vi "FPGA_1R_ADC_1W_DAC_2AI_Jul9.vi"() -> ()   [LabVIEW 2019]
uses:
  <vilib>/rvi/Emulation/niFpgaGetClockAttributes.vi
  <vilib>/rvi/Emulation/niFpgaSctlEmulationGetInTimedLoop.vi
  <vilib>/rvi/Emulation/niFpgaEmulationReportErrorSimple.vi
  <vilib>/rvi/eio/common/nirviEmuTemplateMethod_errors.vi
  <vilib>/rvi/Emulation/niFpgaCriticalErrorInLSC.vi
  <vilib>/eio/EIONode/EIONode.xnode
  <vilib>/rvi/FXPMathLib/basic elements/FxpAddSub/XNode/nifxpmath_AddSub.xnode
  <vilib>/rvi/FXPMathLib/sim/FxpSim.dll
panel:
  out "?":u16(graph)
  out "PD2":u16
  in  "?":bool
  out "PD1":u16
  in  "DAQ stop":bool
  out "ADC Read":bool[](array[boolean])
  out "DAQ TICKS":u32
  in  "DAQ WAIT TICKS":u32=800
  in  "DAC 1 write":bool[](array[boolean])=[FALSE, FALSE, FALSE, FALSE, FALSE, FALSE, FALSE, FALSE, FALSE, FALSE, FALSE, FALSE, FALSE, FALSE, FALSE, FALSE]
  out "XFWD":bool
  out "XREV":bool
  out "YFWD":bool
  out "YREV":bool
  in  "Limit flag stop":bool
  in  "ENC stop":bool
  out "Encoder A Ref":bool
  out "Encoder B Ref":bool
  out "Encoder A":i32
  out "Encoder B":i32
  in  "2^n avg_window":i16=8
  out "ENCODER OVERFLOW":bool
  out "ENCODER TICKS":u32
  in  "ENCODER TICK SETPOINT":u32=8
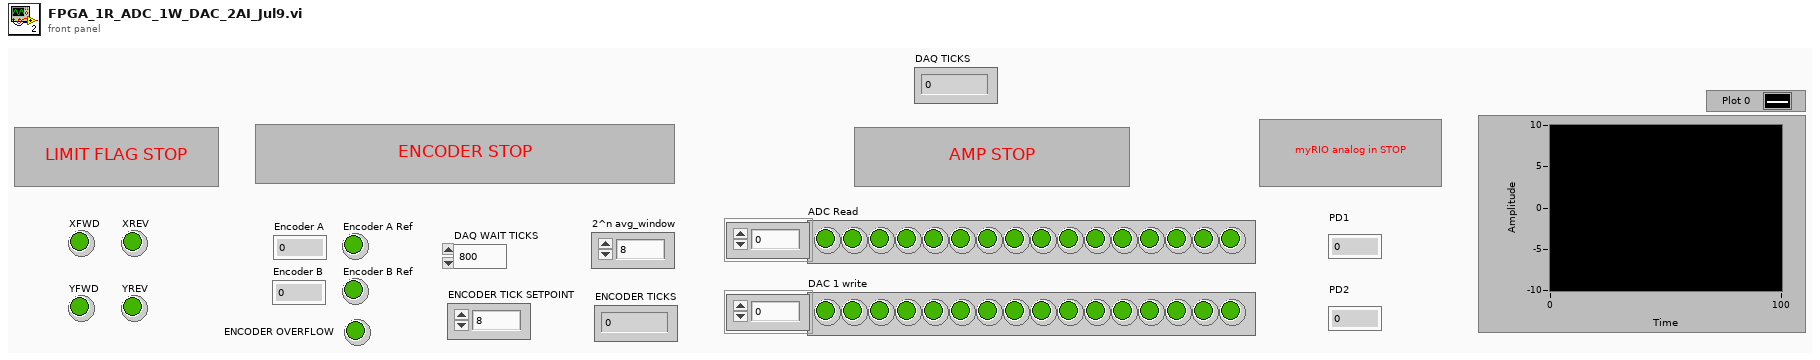
[diagram p1: front panel]
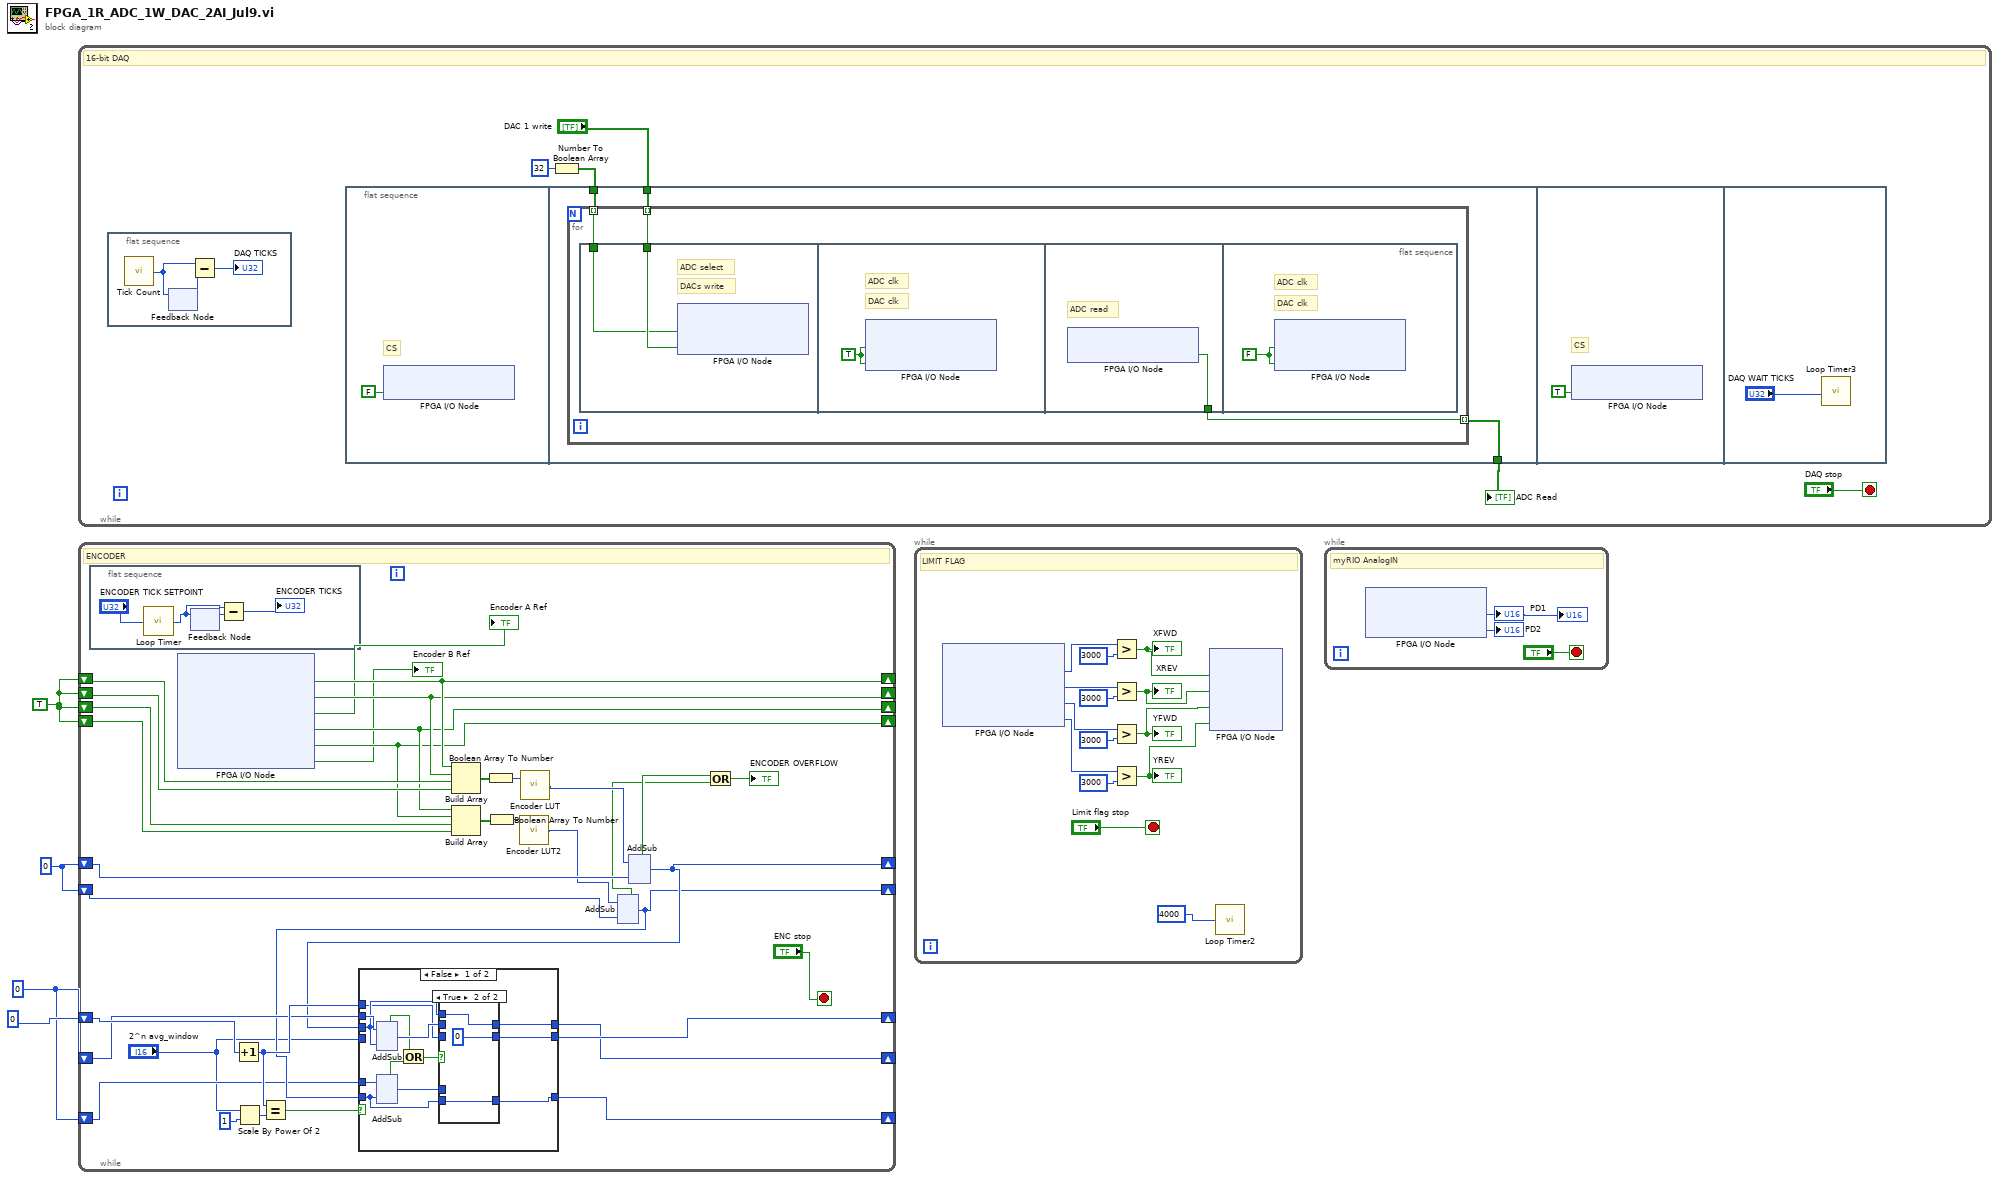
[diagram p0: block diagram]
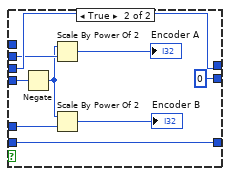
[diagram p3: hidden frame]
diagram:
  w1 = i64 0
  w3 = TRUE
  w4 = 0
  n1 = while {
    stop <- "DAQ stop" stop-if-true
    # "16-bit DAQ"
    n2 = flat-sequence {
      frame #0 {
        n3 = call "Tick Count"() -> ("Tick Count(Ticks)"=w26:u32)
        n4 = feedback #1() -> (w25:u32)  [unwired: 1 in]
        n5 = feedback-in #1(w26) -> ()
        n6 = Subtract(x=w26, y=w25) -> (x-y=→"DAQ TICKS":u32)
      }
    }
    n7 = flat-sequence {
      tunnel: "DAC 1 write" -> [w13]
      tunnel: w7 -> [w12]
      tunnel: [w11] -> w5
      frame #0 {
        # "CS"
        n8 = xnode "FPGA I/O Node"("ConnectorA/DIO4"=FALSE) -> ()  [unwired: 1 in, 1 out]
      }
      frame #1 {
        n9 = for {
          tunnel: w13 -> [w16] mode=indexing
          tunnel: [w15] -> w11 mode=indexing
          tunnel: w12 -> [w14] mode=indexing
          n10 = flat-sequence {
            tunnel: w16 -> [w18]
            tunnel: w14 -> [w17]
            tunnel: [w20] -> w15
            frame #0 {
              # "DACs write"
              # "ADC select"
              n11 = xnode "FPGA I/O Node"("ConnectorA/DIO2"=w17, "ConnectorA/DIO6"=w18) -> ()  [unwired: 2 in, 2 out]
            }
            frame #1 {
              w19 = TRUE ("ConnectorA/DIO3")
              # "DAC clk"
              # "ADC clk"
              n12 = xnode "FPGA I/O Node"("ConnectorA/DIO3"=w19, "ConnectorA/DIO5"=w19) -> ()  [unwired: 2 in, 2 out]
            }
            frame #2 {
              # "ADC read"
              n13 = xnode "FPGA I/O Node"() -> ("ConnectorA/DIO1"=w20:bool)  [unwired: 1 in, 1 out]
            }
            frame #3 {
              w21 = FALSE ("ConnectorA/DIO3")
              # "DAC clk"
              # "ADC clk"
              n14 = xnode "FPGA I/O Node"("ConnectorA/DIO3"=w21, "ConnectorA/DIO5"=w21) -> ()  [unwired: 2 in, 2 out]
            }
          }
        }
      }
      frame #2 {
        # "CS"
        n15 = xnode "FPGA I/O Node"("ConnectorA/DIO4"=TRUE) -> ()  [unwired: 1 in, 1 out]
      }
      frame #3 {
        n16 = call "Loop Timer3"("Count(Ticks)"="DAQ WAIT TICKS") -> ()  [unwired: 1 out]
      }
    }
    n17 = Number To Boolean Array(number=u16 32) -> (Boolean array=w7:bool[])
    "ADC Read" <- w5
  }
  n18 = while {
    shift-right: [w40] -> _
    shift-left: w4 -> [w38]
    shift-right: [w54] -> _
    shift-left: w3 -> [w60]
    shift-right: [w53] -> _
    shift-left: w3 -> [w57]
    shift-right: [w52] -> _
    shift-left: w3 -> [w56]
    shift-right: [w51] -> _
    shift-left: w3 -> [w55]
    shift-right: [w35] -> _
    shift-left: w4 -> [w36]
    shift-right: [w43] -> _
    shift-left: i16 0 -> [w46]
    shift-right: [w42] -> _
    shift-left: w1 -> [w41]
    shift-right: [w34] -> _
    shift-left: w1 -> [w33]
    stop <- "ENC stop" stop-if-true
    # "ENCODER"
    n19 = flat-sequence {
      frame #0 {
        n20 = call "Loop Timer"("Count(Ticks)"="ENCODER TICK SETPOINT") -> ("Tick Count(Ticks)"=w64:u32)
        n21 = feedback #2() -> (w63:u32)  [unwired: 1 in]
        n22 = feedback-in #2(w64) -> ()
        n23 = Subtract(x=w64, y=w63) -> (x-y=→"ENCODER TICKS":u32)
      }
    }
    n24 = xnode "FPGA I/O Node"() -> ("ConnectorA/DIO10"=w54:bool, "ConnectorA/DIO9"=w53:bool, "ConnectorA/DIO11"=→"Encoder A Ref":bool, "ConnectorA/DIO14"=w52:bool, "ConnectorA/DIO13"=w51:bool, "ConnectorA/DIO12"=→"Encoder B Ref":bool)  [unwired: 6 in, 6 out]
    n25 = Increment(x=w46) -> (x+1=w44:i16)
    n26 = Scale By Power Of 2(n="2^n avg_window", x=i64 1) -> (x*2^n=w30:i64)
    n27 = Equal?(x=w44, y=w30) -> (x = y?=w45:bool)
    n28 = Build Array(w54, w53, w60, w57) -> (w58:bool[])
    n29 = Build Array(w52, w51, w56, w55) -> (w59:bool[])
    n30 = Boolean Array To Number(Boolean array=w58) -> (number=w48:u8)
    n31 = Boolean Array To Number(Boolean array=w59) -> (number=w47:u8)
    n32 = call "Encoder LUT2"("address"=w47) -> ("data out"=w37:i32)  [unwired: 8 in]
    n33 = call "Encoder LUT"("address"=w48) -> ("data out"=w39:i32)  [unwired: 8 in]
    n34 = xnode "AddSub"("x"=w37, "y"=w36) -> ("s"=w35:i32, "overflow"=w28:bool)
    n35 = xnode "AddSub"("x"=w39, "y"=w38) -> ("s"=w40:i32, "overflow"=w29:bool)
    n36 = case shown="False" w45 {
      tunnel: w44 -> [w166 _]
      tunnel: [w167 i16 0] -> w43
      tunnel: w40 -> [w170 w288]
      tunnel: [w174 w288] -> w42
      tunnel: w41 -> [w176 w286]
      tunnel: w35 -> [w169 w287]
      tunnel: [w172 w287] -> w34
      tunnel: w33 -> [w175 w283]
      tunnel: "2^n avg_window" -> [_ w285]
      frame False {
        n37 = xnode "AddSub"("x"=w176, "y"=w170) -> ("s"=w173:i64, "overflow"=w165:bool)
        n38 = xnode "AddSub"("x"=w175, "y"=w169) -> ("s"=w171:i64, "overflow"=w164:bool)
        n39 = Or(x=w165, y=w164) -> (x .or. y?=w168:bool)
        n40 = case shown="True" w168 {
          tunnel: [w179 w182] -> w174
          tunnel: w173 -> [w179 _]
          tunnel: [w178 w181] -> w172
          tunnel: w171 -> [w178 _]
          tunnel: w170 -> [_ w182]
          tunnel: w169 -> [_ w181]
          tunnel: [w177 i16 0] -> w167
          tunnel: w166 -> [w177 _]
          frame False {
          }
          frame True {
          }
        }
      }
      frame True {
        n41 = Negate(x=w285) -> (-x=w282:i16)
        n42 = Scale By Power Of 2(n=w282, x=w286) -> (x*2^n=→"Encoder A":i64)
        n43 = Scale By Power Of 2(n=w282, x=w283) -> (x*2^n=→"Encoder B":i64)
      }
    }
    n44 = Or(x=w29, y=w28) -> (x .or. y?=→"ENCODER OVERFLOW":bool)
  }
  n45 = while {
    stop <- "Limit flag stop" stop-if-true
    # "LIMIT FLAG"
    n46 = xnode "FPGA I/O Node"() -> ("ConnectorA/AI0"=w299:u16, "ConnectorA/AI1"=w298:u16, "ConnectorA/AI2"=w297:u16, "ConnectorA/AI3"=w296:u16)  [unwired: 4 in, 4 out]
    n47 = Greater?(x=w299, y=u16 3000) -> (0:w293:bool)
    "XFWD" <- w293
    n48 = Greater?(x=w298, y=u16 3000) -> (0:w292:bool)
    "XREV" <- w292
    n49 = Greater?(x=w297, y=u16 3000) -> (0:w291:bool)
    "YFWD" <- w291
    n50 = Greater?(x=w296, y=u16 3000) -> (0:w290:bool)
    "YREV" <- w290
    n51 = xnode "FPGA I/O Node"("LED0"=w293, "LED1"=w292, "LED2"=w291, "LED3"=w290) -> ()  [unwired: 4 in, 4 out]
    n52 = call "Loop Timer2"("Count(Ticks)"=u32 4000) -> ()  [unwired: 1 out]
  }
  n53 = while {
    stop <- "?" stop-if-true
    # "myRIO AnalogIN"
    n54 = xnode "FPGA I/O Node"() -> ("ConnectorB/AI0"=→"PD1" →"?":u16, "ConnectorB/AI1"=→"PD2":u16)  [unwired: 2 in, 2 out]
  }
